vi "create_square_points.vi"(8 "error in (no error)":errorcluster, 11 "TrajectoryMH100122AODRAPS in":refnum<class "TrajectoryMH100122AODRAPS.lvclass">) -> (0 "error out":errorcluster, 3 "TrajectoryMH100122AODRAPS out":refnum<class "TrajectoryMH100122AODRAPS.lvclass">)   [LabVIEW 2010, in "TrajectoryMH100122AODRAPS.lvclass"]
uses:
  TrajectoryMH100122AODRAPS.lvclass
  common/xcontrols/XImage/XImage/overlays_cluster.ctl
  TrajectoryMH100122AODRAPS.lvclass/TrajectoryMH100122AODRAPS.ctl
  common/xcontrols/XImage/XImage/XImage.xctl
  common/classes/ImageCollection/ImageCollection/ImageCollection.lvclass
  common/classes/Image/Image/Image.lvclass
  class_data.vi
  <vilib>/vision/NI_Vision_Development_Module.lvlib
panel:
  in  "overlay size":i32
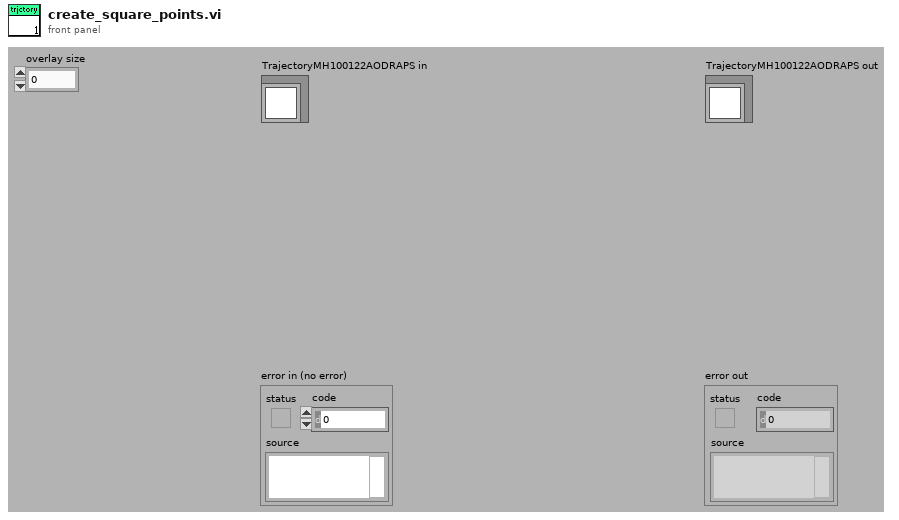
[diagram p1: front panel]
types:
  T1 = typedef "XImage.xctl/overlays_cluster.ctl" = cluster{"overlay array":cluster{i32[][]}[], "overlay name":string, "color (red)":u32, "overlay size":i32, "overlay type":enum16{"crosshair", "circle"}}
  T2 = typedef "ROI Descriptor" = cluster{"Global Rectangle":i32[], "Contours":cluster{"ID":enum32{"External", "Internal"}, "Type":u32, "Coordinates":i32[]}[]}
  T3 = cluster{"Global Rectangle":i32[], "Contours":cluster{"Contour Type":u32, "ROI Type":u32, "Points":i32[]}[]}
  T4 = cluster{"Global Rectangle":i32[], "Contours":cluster{"Contour Type":u32, "ROI Type":u32, "Points":i32[]}[]}[]
  T5 = cluster{"Contour Type":u32, "ROI Type":u32, "Points":i32[]}[]
  T6 = typedef "IMAQ Image.ctl" = refnum<image>
  T7 = typedef "IMAQ Rectangle" = cluster{"Left":i32, "Top":i32, "Right":i32, "Bottom":i32, "Rotation":dbl}
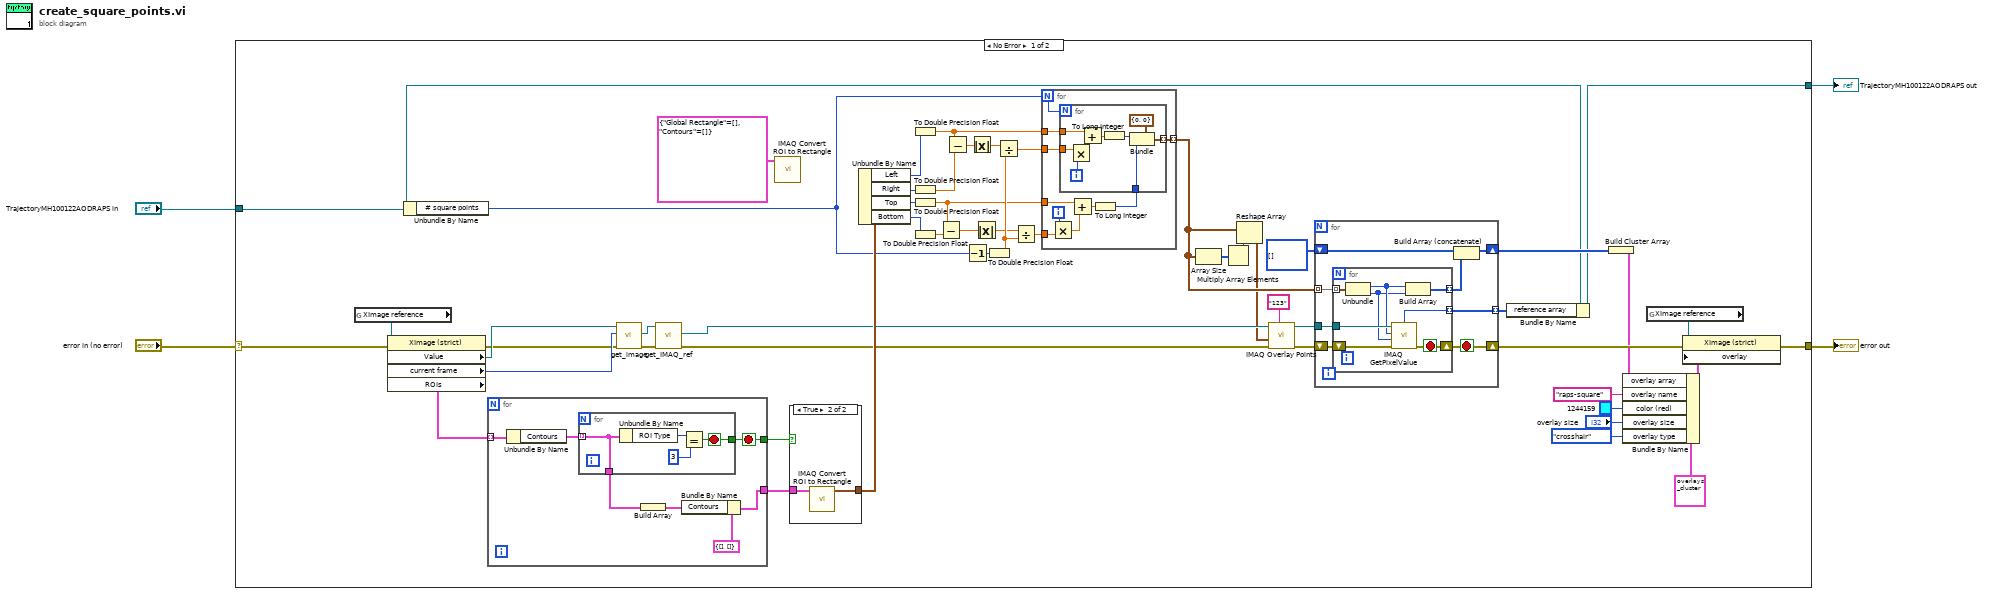
[diagram p0: block diagram]
diagram:
  n1 = case shown="No Error" "error in (no error)" {
    selector: "error in (no error)" -> [w24 w106]
    tunnel: [w17 w106] -> w3
    tunnel: [w5 w105] -> w1
    tunnel: "TrajectoryMH100122AODRAPS in" -> [w6 w105]
    frame No Error {
      n2 = global read "class_data.vi" "XImage reference"() -> (w25:refnum<vi>)
      n3 = property on="Property Node" class="XImage (strict)"(reference=w25, error in=w24) -> (error out=w21:errorcluster, "Value"=w23:refnum<class "ImageCollection.lvclass">, "current frame"=w31:i32, "ROIs"=w56:T4)  [unwired: 1 out]
      n4 = Unbundle By Name(w6) -> ("# square points"=w26:i32)
      n5 = for {
        tunnel: w56 -> [w99] mode=indexing
        tunnel: [w94] -> w54
        tunnel: [w100] -> w53
        stop <- w100 stop-if-true
        n6 = Unbundle By Name(w99) -> ("Contours"=w97:T5)
        n7 = for {
          tunnel: w97 -> [w101] mode=indexing
          tunnel: [w102] -> w100
          tunnel: [w101] -> w96
          stop <- w102 stop-if-true
          n8 = Unbundle By Name(w101) -> ("ROI Type"=w104:u32)
          n9 = Equal?(x=w104, y=u32 3) -> (x = y?=w102:bool)
        }
        n10 = Build Array(w96) -> (w95:T5)
        n11 = Bundle By Name(cluster=T3 {"Global Rectangle"=[], "Contours"=[]} ("ROI"), "Contours"=w95) -> (w94:T3)
      }
      n12 = call-dynamic "get_image.vi"("error in (no error)"=w21, "index"=w31, "ImageCollection in"=w23) -> ("error out"=w22:errorcluster, "Image.lvclass"=w30:refnum<class "Image.lvclass">)  [unwired: 6 in, 1 out]
      n13 = call-dynamic "get_IMAQ_ref.vi"("error in (no error)"=w22, "Image.lvclass in"=w30) -> ("error out"=w20:errorcluster, "Image"=w29:T6)  [unwired: 5 in, 3 out]
      n14 = call "IMAQ Convert ROI to Rectangle"("ROI Descriptor"=T2 {"Global Rectangle"=[], "Contours"=[]}) -> ()  [unwired: 8 in, 2 out]
      n15 = case shown="True" w53 {
        tunnel: w54 -> [_ w93]
        tunnel: [_ w92] -> w34
        frame False {
        }
        frame True {
          n16 = call "IMAQ Convert ROI to Rectangle"("ROI Descriptor"=w93) -> ("Rectangle"=w92:T7)  [unwired: 8 in, 1 out]
        }
      }
      n17 = Unbundle By Name(w34) -> ("Left"=w38:i32, "Right"=w39:i32, "Top"=w37:i32, "Bottom"=w46:i32)
      n18 = To Double Precision Float(number=w38) -> (double precision float=w43:dbl)
      n19 = To Double Precision Float(number=w39) -> (double precision float=w45:dbl)
      n20 = To Double Precision Float(number=w37) -> (double precision float=w47:dbl)
      n21 = To Double Precision Float(number=w46) -> (double precision float=w48:dbl)
      n22 = Subtract(x=w47, y=w48) -> (x-y=w49:dbl)
      n23 = Subtract(x=w43, y=w45) -> (x-y=w40:dbl)
      n24 = Decrement(x=w26) -> (x-1=w41:i32)
      n25 = Absolute Value(x=w40) -> (abs(x)=w44:dbl)
      n26 = Absolute Value(x=w49) -> (abs(x)=w50:dbl)
      n27 = To Double Precision Float(number=w41) -> (double precision float=w51:dbl)
      n28 = Divide(x=w44, y=w51) -> (x/y=w42:dbl)
      n29 = Divide(x=w50, y=w51) -> (x/y=w52:dbl)
      n30 = for {
        N: w26 -> [w76]
        tunnel: w42 -> [w82]
        tunnel: w43 -> [w74]
        tunnel: [w81] -> w28 mode=indexing
        tunnel: w52 -> [w79]
        tunnel: w47 -> [w75]
        i -> [w80]
        n31 = Multiply(x=w80, y=w79) -> (x*y=w78:dbl)
        n32 = Add(x=w75, y=w78) -> (x+y=w77:dbl)
        n33 = To Long Integer(number=w77) -> (32bit integer=w73:i32)
        n34 = for {
          N: w76 -> [_]
          tunnel: w82 -> [w88]
          tunnel: w74 -> [w90]
          tunnel: [w85] -> w81 mode=indexing
          tunnel: w73 -> [w84]
          i -> [w87]
          n35 = Multiply(x=w88, y=w87) -> (x*y=w86:dbl)
          n36 = Add(x=w90, y=w86) -> (x+y=w89:dbl)
          n37 = To Long Integer(number=w89) -> (32bit integer=w83:i32)
          n38 = Bundle(cluster=cluster{"X":i32, "Y":i32} {"X"=0, "Y"=0} ("Point Coordinates"), "X"=w83, "Y"=w84) -> (w85:cluster{"X":i32, "Y":i32})
        }
      }
      n39 = Array Size(array=w28) -> (size(s)=w35:i32[])
      n40 = Multiply Array Elements(1:w35) -> (0:w36:i32)
      n41 = Reshape Array(w28, w36) -> (w27:cluster{"X":i32, "Y":i32}[])
      n42 = call "IMAQ Overlay Points"("Group"="123", "Array of Points"=w27, "Image"=w29) -> ("Image Out"=w33:T6)  [unwired: 7 in, 1 out]
      n43 = for {
        tunnel: w33 -> [w64]
        shift-right: [w60] -> w18
        shift-left: w20 -> [w63]
        tunnel: w28 -> [w62] mode=indexing
        tunnel: [w61] -> w7 mode=indexing
        shift-right: [w58] -> w8
        shift-left: i32[][] [] -> [w59]
        stop <- w60 stop-if-true
        n44 = for {
          tunnel: w64 -> [w72]
          shift-right: [w68] -> w60
          shift-left: w63 -> [w71]
          tunnel: w62 -> [w70] mode=indexing
          tunnel: [w69] -> w61 mode=indexing
          tunnel: [w65] -> w57 mode=indexing
          stop <- w68 stop-if-true
          n45 = Unbundle(w70) -> ("X"=w67:i32, "Y"=w66:i32)
          n46 = call "IMAQ GetPixelValue"("Image"=w72, "X Coordinate"=w67, "Y Coordinate"=w66, "error in (no error)"=w71) -> ("Pixel Value (U16)"=w69:u16, "error out"=w68:errorcluster)  [unwired: 2 in, 3 out]
          n47 = Build Array(w67, w66) -> (w65:i32[])
        }
        n48 = Build Array (concatenate)(w59, w57) -> (w58:i32[][])
      }
      n49 = Bundle By Name(cluster=w6, "reference array"=w7) -> (w5:refnum<class "TrajectoryMH100122AODRAPS.lvclass">)
      n50 = Build Cluster Array(w8) -> (w14:cluster{i32[][]}[])
      n51 = Bundle By Name(cluster=T1 {"overlay array"=[], "overlay name"="", "color (red)"=16711680, "overlay size"=0, "overlay type"=enum."crosshair"} ("Overlay"), "overlay array"=w14, "overlay name"="raps-square", "color (red)"=u32 1244159, "overlay size"="overlay size", "overlay type"=enum16{"crosshair", "circle"}."crosshair") -> (w15:T1)
      n52 = global read "class_data.vi" "XImage reference"() -> (w19:refnum<vi>)
      n53 = property on="Property Node" class="XImage (strict)"(reference=w19, error in=w18, "overlay"=w15) -> (error out=w17:errorcluster)  [unwired: 1 out]
    }
    frame Error {
    }
  }
  "error out" <- w3
  "TrajectoryMH100122AODRAPS out" <- w1
